vi "EAGLE Main.vi"   [LabVIEW 2015]
uses:
  Host Globals.vi
panel:
  # "EAGLE"
  # "External Automatic Glaucoma Laser"
  # "Revision: 2017r1"
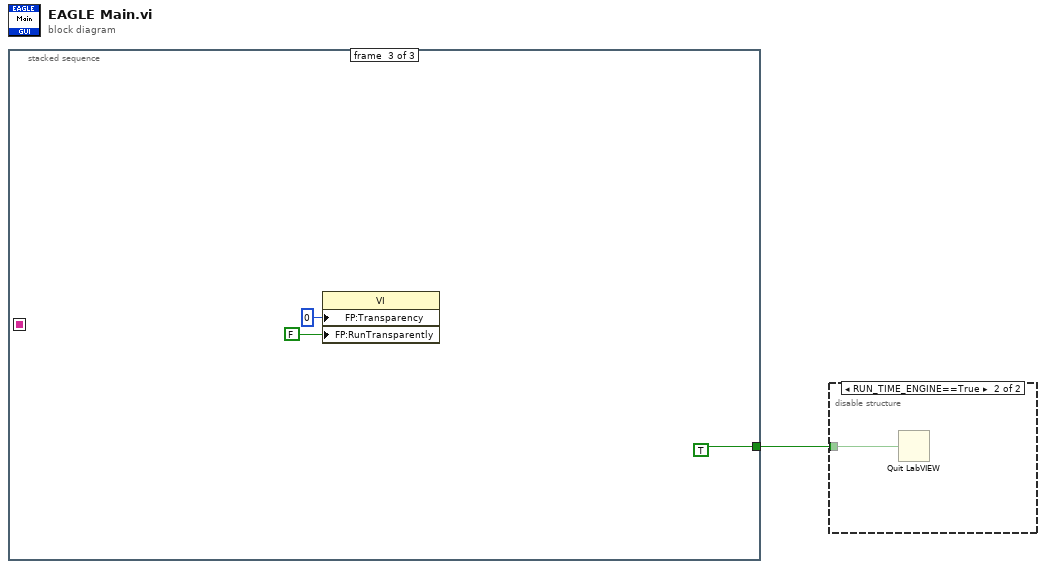
[diagram p0: block diagram]
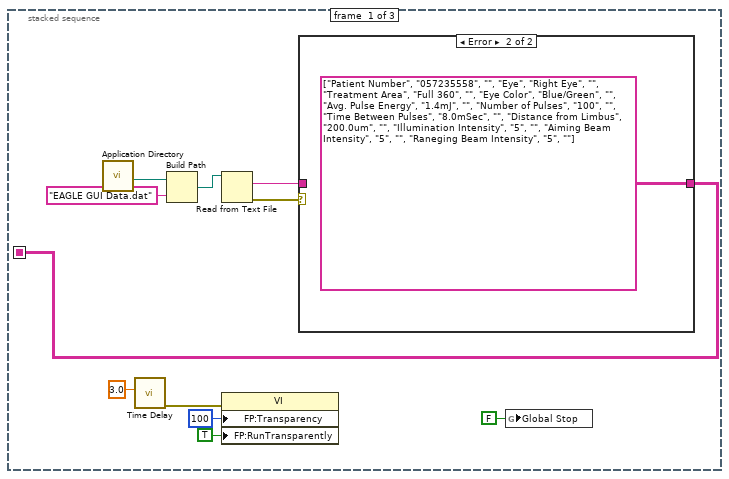
[diagram p3: hidden frame]
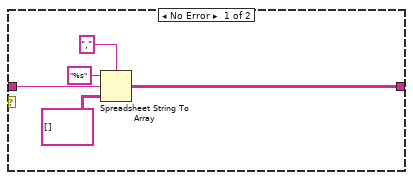
[diagram p4: hidden frame]
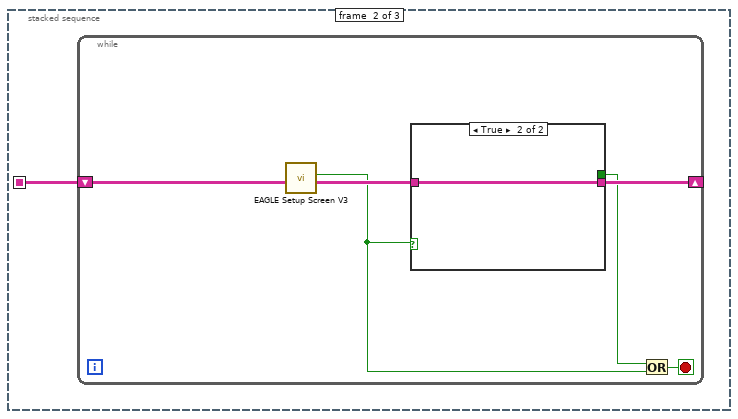
[diagram p5: hidden frame]
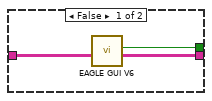
[diagram p6: hidden frame]
diagram:
  n1 = stacked-sequence {
    seq-local: [w7 _ _] -> [_ w19 _]
    tunnel: [_ _ TRUE] -> w1
    frame #0 {
      n2 = call <vilib>:"Application Directory.vi"() -> ("Application Directory"=w12:path)
      n3 = call "Time Delay"("Delay Time (s)"=3.0) -> ("error out"=w6:errorcluster)  [unwired: 10 in]
      n4 = Build Path(base path=w12, name or relative path="EAGLE GUI Data.dat") -> (appended path=w10:path)
      n5 = Read from Text File(file (use dialog)=w10) -> (text=w9:string, error out=w8:errorcluster)  [unwired: 3 in, 2 out]
      n6 = property class="VI"(error in=w6, "FP:Transparency"=u8 100 ("Front Panel Window:Transparency"), "FP:RunTransparently"=TRUE ("Front Panel Window:Run VI Transparently")) -> ()  [unwired: 1 in, 2 out]
      n7 = case shown="Error" w8 {
        tunnel: w9 -> [w17 _]
        tunnel: [w13 string[][] [["Patient Number", "057235558", ""], ["Eye", "Right Eye", ""], ["Treatment Area", "Full 360", ""], ["Eye Color", "Blue/Green", ""], ["Avg. Pulse Energy", "1.4mJ", ""], ["Number of Pulses", "100", ""], ["Time Between Pulses", "8.0mSec", ""], ["Distance from Limbus", "200.0um", ""], ["Illumination Intensity", "5", ""], ["Aiming Beam Intensity", "5", ""], ["Raneging Beam Intensity", "5", ""]]] -> w7
        frame No Error {
          n8 = Spreadsheet String To Array(delimiter (Tab)=",", format string="%s", spreadsheet string=w17, array type (2D Dbl)=string[][] []) -> (array=w13:string[][])
        }
        frame Error {
        }
      }
      n9 = global write "Host Globals.vi" "Global Stop"(FALSE ("Global Stop")) -> ()
    }
    frame #1 {
      n10 = while {
        shift-right: [w25] -> _
        shift-left: w19 -> [w24]
        stop <- w22 stop-if-true
        n11 = call "EAGLE Setup Screen V3.vi"("TableIn"=w24) -> ("TableOut"=w23:string[][], "Exit"=w20:bool)  [unwired: 9 in]
        n12 = case shown="True" w20 {
          tunnel: w23 -> [w28 w29]
          tunnel: [w27 w29] -> w25
          tunnel: [w26 _] -> w21
          frame False {
            n13 = call "EAGLE GUI V6.vi"("TableIn"=w28) -> ("GUI Table"=w27:string[][], "Exit"=w26:bool)  [unwired: 9 in]
          }
          frame True {
          }
        }
        n14 = Or(x=w21, y=w20) -> (x .or. y?=w22:bool)
      }
    }
    frame #2 {
      n15 = property class="VI"("FP:Transparency"=u8 0 ("Front Panel Window:Transparency"), "FP:RunTransparently"=FALSE ("Front Panel Window:Run VI Transparently")) -> ()  [unwired: 2 in, 2 out]
    }
  }
  n16 = disable-structure shown="RUN_TIME_ENGINE==True" {
    disable-tunnel: w1 -> [_ w33]
    frame condition #0 (active) {
    }
    frame condition #1 {
      n17 = Quit LabVIEW(quit? (T)=w33) -> ()
    }
  }
